vi "Clear Calculate Data.vi"(8 "error in (no error)":errorcluster, 10 "Clear Operation (0: Clear All)":i32(ring) items=["Clear All", "Clear Statistical Data", "Clear Limit Data", "Clear Histogram Data"], 11 "VISA resource name":refnum<visa-resource-name>) -> (0 "error out":errorcluster, 3 "VISA resource name out":refnum<visa-resource-name>)   [LabVIEW 2020, in "Agilent 3446X Series.lvlib"]
doc: "Clears the calculation data.\n\n<b>Note(s):</b>\nThis vi is not supported for EDU34450A model."
uses:
  <instrlib>/Agilent 3446X Series/Agilent 3446X Series.lvlib
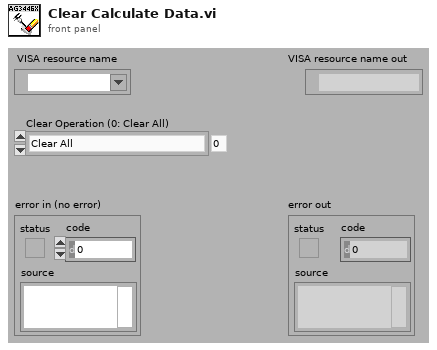
[diagram p1: front panel]
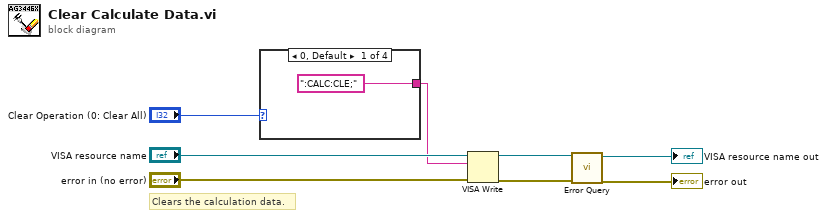
[diagram p0: block diagram]
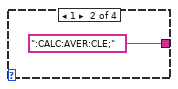
[diagram p2: hidden frame]
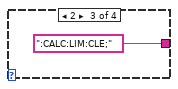
[diagram p3: hidden frame]
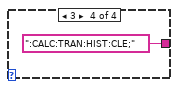
[diagram p4: hidden frame]
diagram:
  # "Clears the calculation data."
  n1 = case shown="0, Default" "Clear Operation (0: Clear All)" {
    tunnel: [":CALC:CLE;" ("write buffer") ":CALC:AVER:CLE;" ("write buffer") ":CALC:LIM:CLE;" ("write buffer") ":CALC:TRAN:HIST:CLE;" ("write buffer")] -> w1
    frame 0, Default {
    }
    frame 1 {
    }
    frame 2 {
    }
    frame 3 {
    }
  }
  n2 = VISA Write(VISA resource name="VISA resource name", write buffer=w1, error in (no error)="error in (no error)") -> (VISA resource name out=w4:refnum<visa-resource-name>, error out=w3:errorcluster)  [unwired: 1 out]
  n3 = call <instrlib>:"Error Query.vi"("error in (no error)"=w3, "VISA resource name"=w4) -> ("error out"=→"error out":errorcluster, "VISA resource name out"=→"VISA resource name out":refnum<visa-resource-name>)  [unwired: 8 out]
